vi "Diode test.vi"() -> ()   [LabVIEW 2016]
uses:
  <vilib>/DAQmx/create/channels.llb/DAQmx Create Channel (AI-Voltage-Basic).vi
panel:
  out "Waveform Graph":dbl[][](graph)
  in  "stop (F)":bool
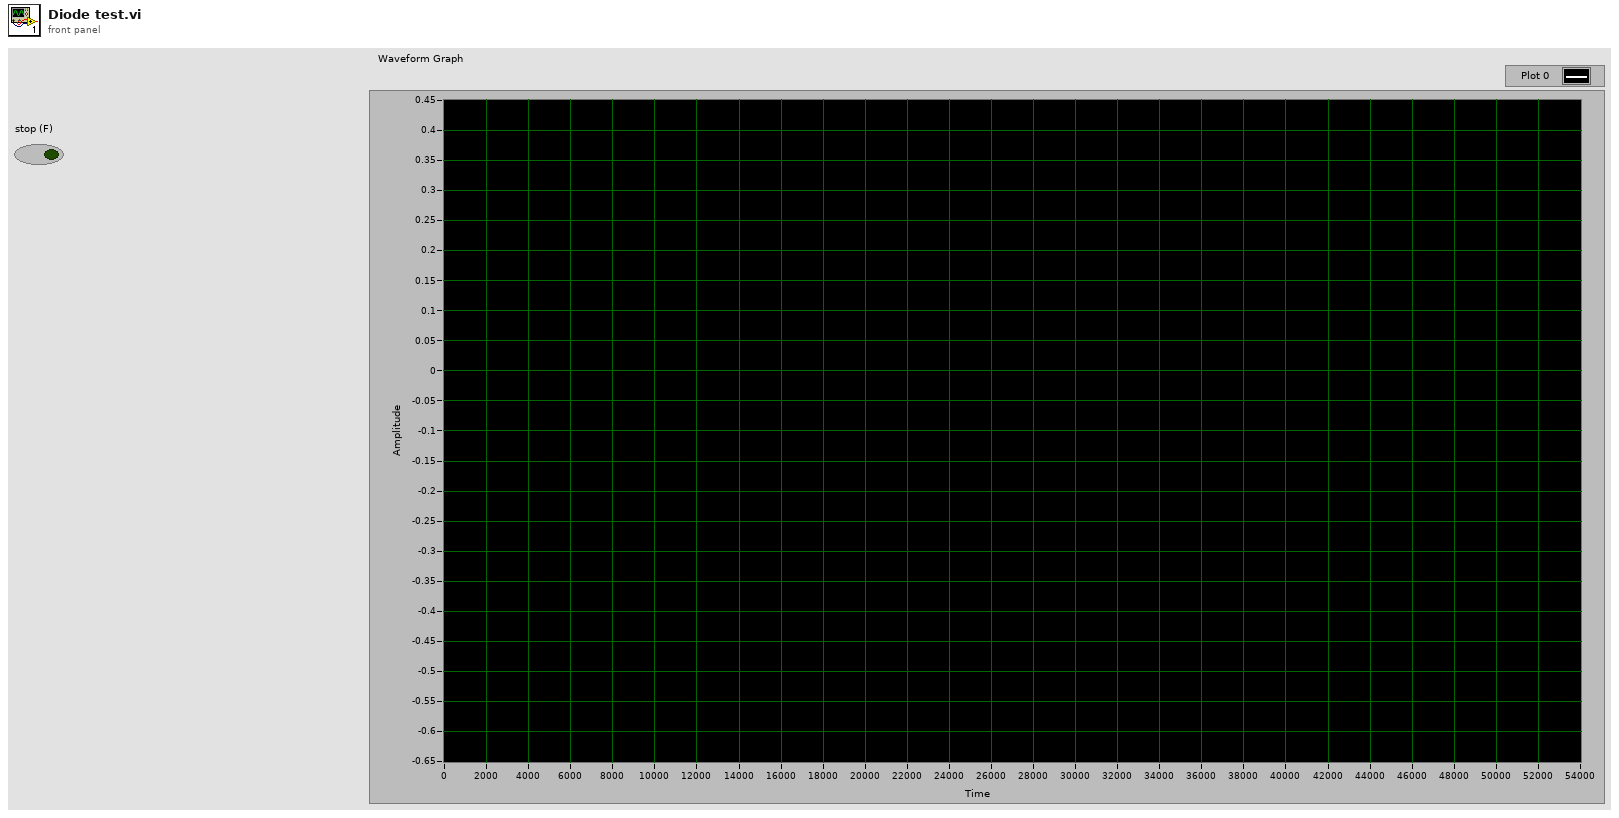
[diagram p1: front panel]
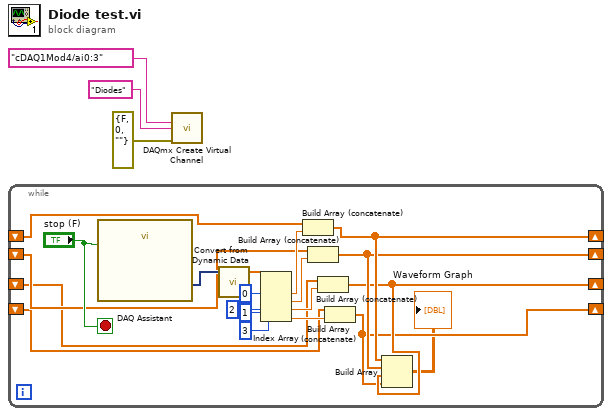
[diagram p0: block diagram]
diagram:
  n1 = while {
    shift-right: [w8] -> _
    shift-left: _ -> [w22]
    shift-right: [w7] -> _
    shift-left: _ -> [w11]
    shift-right: [w6] -> _
    shift-left: _ -> [w10]
    shift-right: [w5] -> _
    shift-left: _ -> [w9]
    stop <- "stop (F)" stop-if-true
    n2 = call "DAQ Assistant"("stop (T)"="stop (F)") -> ("data"=w21:dynamicdata)  [unwired: 16 in, 2 out]
    n3 = call "Convert from Dynamic Data"("Dynamic Data Type"=w21) -> ("Array"=w20:dbl[])  [unwired: 3 in]
    n4 = Index Array(array=w20, index #1=0 ("index"), index #2=1 ("index"), index #3=2 ("index"), index #4=3 ("index")) -> (element #1=w15:dbl, element #2=w14:dbl, element #3=w13:dbl, element #4=w12:dbl)
    n5 = Build Array (concatenate)(w22, w15) -> (w8:dbl[])
    n6 = Build Array (concatenate)(w11, w14) -> (w7:dbl[])
    n7 = Build Array (concatenate)(w10, w13) -> (w6:dbl[])
    n8 = Build Array (concatenate)(w9, w12) -> (w5:dbl[])
    n9 = Build Array(w8, w7, w6, w5) -> (→"Waveform Graph":dbl[][])
  }
  n10 = call-poly <vilib>:"DAQmx Create Virtual Channel.vi"("physical channels"=tag "cDAQ1Mod4/ai0:3", "name to assign"="Diodes", "error in"=errorcluster {"status"=FALSE, "code"=0, "source"=""}) -> ()  [unwired: 11 in, 2 out]
